vi "2.设置名称.vi"(8 "error in":errorcluster, 9 "SavePath":path, 10 "Name":string, 11 "Module ID":i32=-1) -> (0 "error out":errorcluster, 1 "OK":bool, 3 "Module ID Out":i32=-1)   [LabVIEW 2020, in "PichartInterface.lvlib"]
uses:
  PichartInterface.lvlib
  <vilib>/DD/DDToolsVIPM/PieChartInterface/PieChart.lvlibp
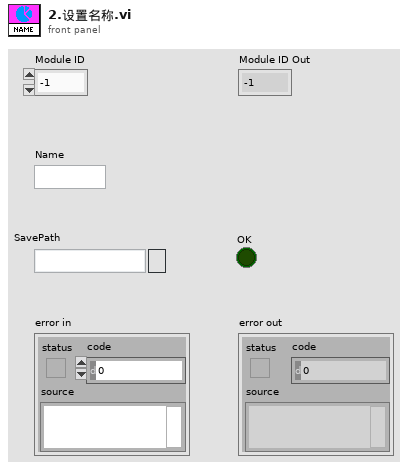
[diagram p1: front panel]
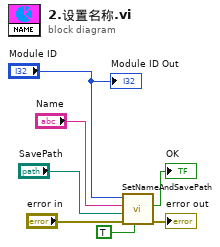
[diagram p0: block diagram]
diagram:
  n1 = call <vilib>:"SetNameAndSavePath.vi"("wait for reply (T)"=TRUE, "error in"="error in", "SavePath"="SavePath", "Name"="Name", "Module ID"="Module ID") -> ("error out"=→"error out":errorcluster, "OK"=→"OK":bool)  [unwired: 4 in, 1 out]
  "Module ID Out" <- "Module ID"
